vi "Nadaj nazwy AI DI.vi"(4 "DI opisy in":string[](array[string]), 6 "AI opisy in":string[](array[string]), 8 "error in (no error)":errorcluster, 10 "Kanaly in":T1) -> (0 "error out":errorcluster, 2 "Kanaly out":T1)   [LabVIEW 2014]
doc: "Nadaje nazwy aktywnym kanałom AI oraz DI\nna podstawie GUI\nWłaściwości:\n- NI_ChannelName - nazwa wykresu\n- NI_UnitDescription - jednostka (cyfrowa \"Dig\")"
uses:
  Kontrolki/Przetwarzanie/Kanaly.ctl
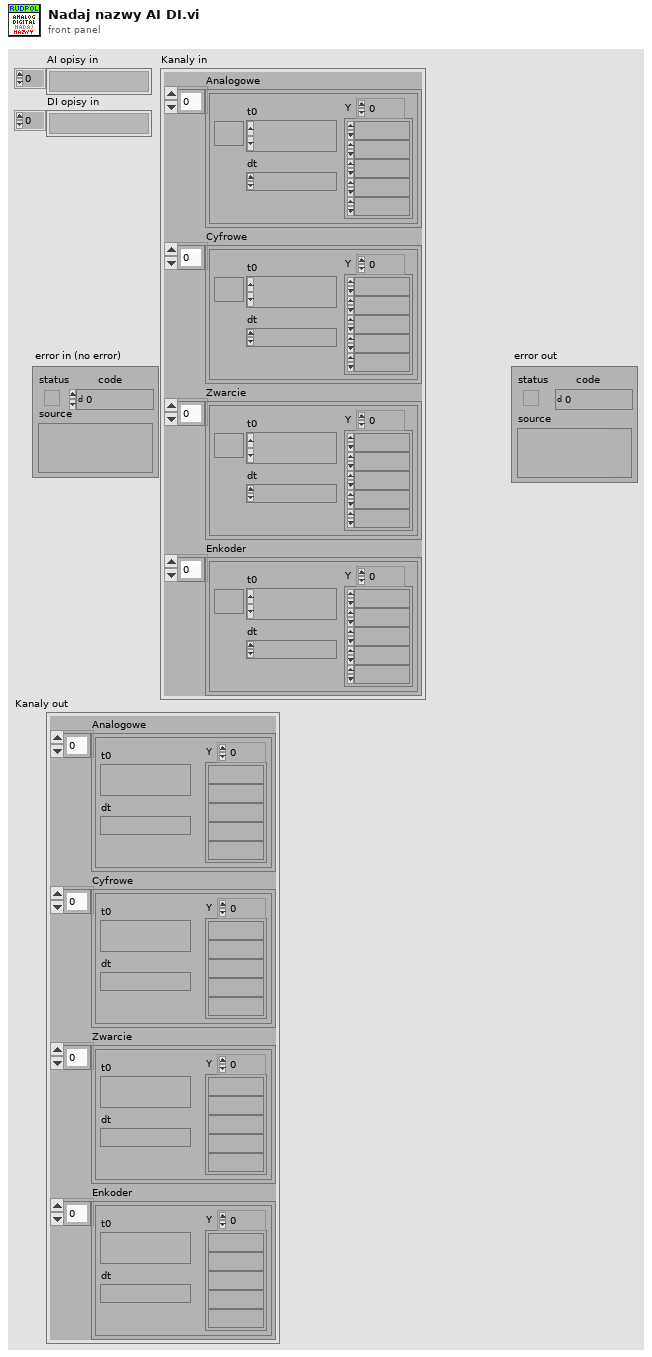
[diagram p1: front panel]
types:
  T1 = typedef "Kanaly.ctl" = cluster{"Analogowe":waveform(dbl)[], "Cyfrowe":waveform(dbl)[], "Zwarcie":waveform(dbl)[], "Enkoder":waveform(dbl)[]}
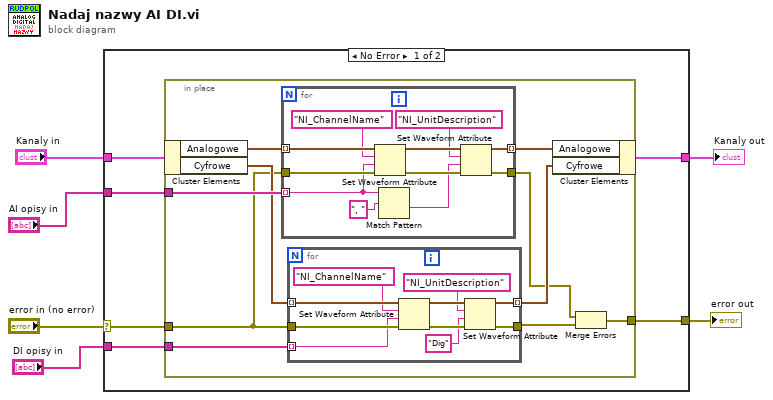
[diagram p0: block diagram]
diagram:
  n1 = case shown="No Error" "error in (no error)" {
    selector: "error in (no error)" -> [w11 w45]
    tunnel: [w10 w45] -> w5
    tunnel: "Kanaly in" -> [w12 w44]
    tunnel: [w7 w44] -> w3
    tunnel: "AI opisy in" -> [w9 _]
    tunnel: "DI opisy in" -> [w8 _]
    frame No Error {
      n2 = in-place {
        in-place-border: w11 -> [w18]
        in-place-border: [w13] -> w10
        in-place-border: w9 -> [w20]
        in-place-border: w8 -> [w17]
        n3 = in-place-cluster #1(w12) -> ("Analogowe"=w22:waveform(dbl)[], "Cyfrowe"=w19:waveform(dbl)[])
        n4 = for {
          tunnel: w22 -> [w43] mode=indexing
          tunnel: [w34] -> w21 mode=indexing
          tunnel: w18 -> [w41]
          tunnel: [w35] -> w14
          tunnel: w20 -> [w40] mode=indexing
          n5 = Set Waveform Attribute(4:w41, 5:w40, 6:"NI_ChannelName" ("name"), 7:w43) -> (0:w37:errorcluster, 3:w38:waveform(dbl))  [unwired: 1 out]
          n6 = Match Pattern(string=w40, regular expression=", ") -> (after substring=w36:string)  [unwired: 1 in, 3 out]
          n7 = Set Waveform Attribute(4:w37, 5:w36, 6:"NI_UnitDescription" ("name"), 7:w38) -> (0:w35:errorcluster, 3:w34:waveform(dbl))  [unwired: 1 out]
        }
        n8 = for {
          tunnel: w19 -> [w32] mode=indexing
          tunnel: [w25] -> w16 mode=indexing
          tunnel: w18 -> [w30]
          tunnel: [w28] -> w15
          tunnel: w17 -> [w29] mode=indexing
          n9 = Set Waveform Attribute(4:w30, 5:w29, 6:"NI_ChannelName" ("name"), 7:w32) -> (0:w27:errorcluster, 3:w26:waveform(dbl))  [unwired: 1 out]
          n10 = Set Waveform Attribute(4:w27, 5:"Dig" ("name"), 6:"NI_UnitDescription" ("name"), 7:w26) -> (0:w28:errorcluster, 3:w25:waveform(dbl))  [unwired: 1 out]
        }
        n11 = in-place-cluster #1("Analogowe"=w21, "Cyfrowe"=w16) -> (w7:T1)
        n12 = Merge Errors(w14, w15) -> (w13:errorcluster)
      }
    }
    frame Error {
    }
  }
  "error out" <- w5
  "Kanaly out" <- w3
